vi "FM Voice Receiver.vi"() -> ()   [LabVIEW 2013]
uses:
  <vilib>/sound2/lvsound2.llb/Sound Output Write (DBL).vi
  <instrlib>/niUSRP/niUSRP Fetch Rx Data (CDB WDT).vi
  <vilib>/Analysis/2dsp.llb/Rational Resample (single channel, DBL).vi
  <vilib>/express/express analysis/Spectral/Block/exnSpectralBlock spectral measurements RMS poly.vi
  <vilib>/express/express analysis/Spectral/Block/exnSpectralBlock spectral measurements RMS WFM.vi
  <vilib>/express/express analysis/Spectral/XNode/ExpressSpectralMeasurementsBlockNode.xnode
  <vilib>/Analysis/NI_AALPro.lvlib
panel:
  out "File Error Out":errorcluster
  in  "Sound Format":T1={"sample rate (S/s)"=44100.0, "number of channels"=1.0, "bits per sample"=16.0}
  out "Spectrum (FFT)":cluster{"f0":dbl, "df":dbl, "magnitude":dbl[]}(graph)
  out "Waveform":waveform(dbl)(graph)
  out "Constellation":cluster{dbl[], dbl[]}(graph)
  out "USRP Error Out":errorcluster
  out "Coerced Gain":dbl format="%#_6f"
  out "Coerced Carrier Freq.":dbl=2400010000.007024 format="%#_6p"
  out "Coerced IQ Rate":dbl=200000.0 format="%#_6p"
  in  "Stop":bool
  in  "Active Antenna":string="RX2"
  in  "Gain":dbl format="%#_6f"
  in  "Carrier Frequency":dbl=1200000000.0 format="%#_6p"
  in  "IQ Rate":dbl=200000.0 format="%#_6p"
  in  "Device Address":refnum<k15>="192.168.10.2"
  in  "Number of Samples":i32=44100
  # "FM Receiver"
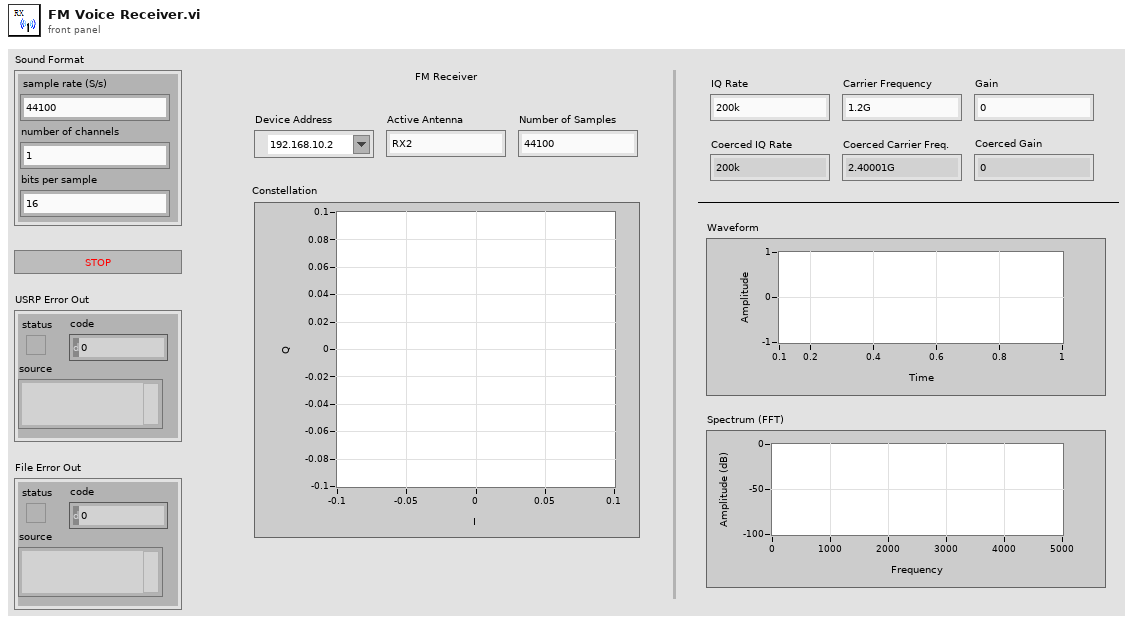
[diagram p1: front panel]
types:
  T1 = cluster{"sample rate (S/s)":dbl, "number of channels":dbl, "bits per sample":dbl}
  T2 = typedef "Sound Output Task ID.ctl" = u32
  T3 = cluster{"averaging mode":u16, "weighting mode":u16, "number of averages":u32}
  T4 = cluster{"dB On (F)":bool, "unwrap phase (F)":bool, "convert to degree (F)":bool}
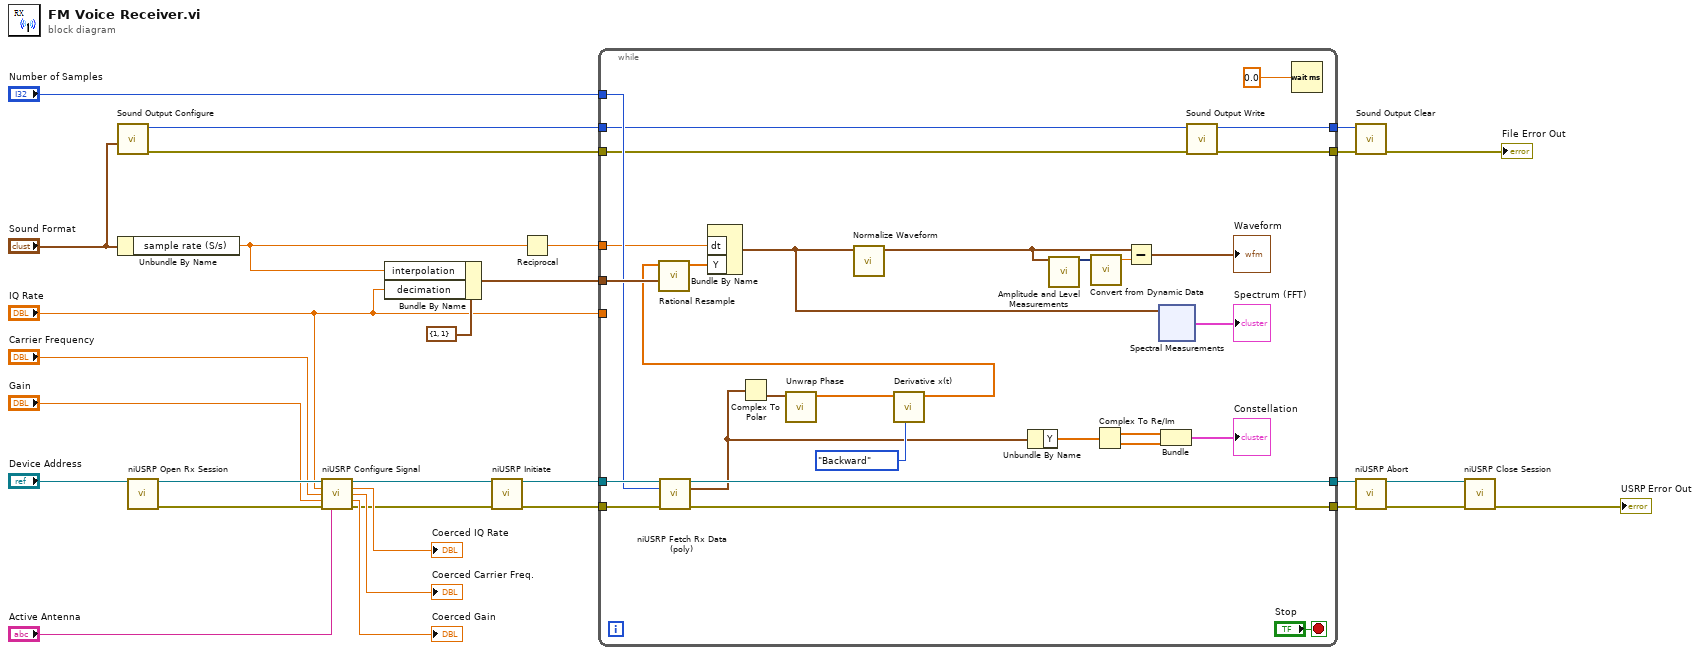
[diagram p0: block diagram]
diagram:
  n1 = call <vilib>:"Sound Output Configure.vi"("sound format"="Sound Format") -> ("error out"=w4:errorcluster, "task ID"=w5:T2)  [unwired: 9 in]
  n2 = Unbundle By Name("Sound Format") -> ("sample rate (S/s)"=w12:dbl)
  n3 = call <instrlib>:"niUSRP Open Rx Session.vi"("device names"="Device Address") -> ("session handle out"=w30:refnum<k15>, "error out"=w29:errorcluster)  [unwired: 13 in]
  n4 = call <instrlib>:"niUSRP Configure Signal.vi"("session handle"=w30, "IQ rate"="IQ Rate", "carrier frequency"="Carrier Frequency", "gain"="Gain", "error in (no error)"=w29, "active antenna"="Active Antenna") -> ("session handle out"=w16:refnum<k15>, "coerced IQ rate"=→"Coerced IQ Rate":dbl, "coerced carrier frequency"=→"Coerced Carrier Freq.":dbl, "coerced gain"=→"Coerced Gain":dbl, "error out"=w14:errorcluster)  [unwired: 5 in]
  n5 = Bundle By Name(cluster=cluster{"decimation":i32, "interpolation":i32} {"decimation"=1, "interpolation"=1}, "interpolation"=w12, "decimation"="IQ Rate") -> (w24:cluster{"decimation":i32, "interpolation":i32})
  n6 = call <instrlib>:"niUSRP Initiate.vi"("session handle"=w16, "error in (no error)"=w14) -> ("session handle out"=w15:refnum<k15>, "error out"=w13:errorcluster)  [unwired: 12 in]
  n7 = Reciprocal(x=w12) -> (1/x=w7:dbl)
  n8 = while {
    tunnel: w15 -> [w59]
    tunnel: [w57] -> w11
    tunnel: [w56] -> w10
    tunnel: w13 -> [w55]
    tunnel: "Number of Samples" -> [w51]
    tunnel: w24 -> [w54]
    tunnel: "IQ Rate" -> [_]
    tunnel: w7 -> [w45]
    tunnel: w5 -> [w40]
    tunnel: w4 -> [w39]
    tunnel: [w38] -> w3
    tunnel: [w37] -> w2
    stop <- "Stop" stop-if-true
    n9 = call-poly <instrlib>:"niUSRP Fetch Rx Data (poly).vi"("session handle"=w59, "number of samples"=w51, "error in (no error)"=w55) -> ("session handle out"=w57:refnum<k15>, "data"=w36:waveform(cdb), "error out"=w56:errorcluster)  [unwired: 9 in, 1 out]
    n10 = Complex To Polar(r * e^(i*theta)=w36) -> (theta=w44:waveform(dbl))  [unwired: 1 out]
    n11 = call <vilib>:"Unwrap Phase.vi"("Phase"=w44) -> ("Unwrapped Phase"=w43:dbl[])  [unwired: 9 in, 1 out]
    n12 = call <vilib>:"Derivative x(t).vi"("method"=enum16{"Backward"}."Backward", "X"=w43) -> ("dX/dt"=w41:dbl[])  [unwired: 8 in, 1 out]
    n13 = call-poly <vilib>:"Rational Resample.vi"("resample factor"=w54, "X"=w41) -> ("Y"=w46:dbl[])  [unwired: 7 in, 2 out]
    n14 = Bundle By Name("dt"=w45, "Y"=w46) -> (w32:waveform(dbl))  [unwired: 1 in]
    n15 = call <vilib>:"Normalize Waveform.vi"("waveform in"=w32) -> ("normalized waveform"=w35:waveform(dbl))  [unwired: 7 in, 3 out]
    n16 = Unbundle By Name(w36) -> ("Y"=w48:cdb[])
    n17 = call "Amplitude and Level Measurements"("Signals"=w35) -> ("Mean (DC)"=w34:dynamicdata)  [unwired: 13 in, 1 out]
    n18 = call "Convert from Dynamic Data"("Dynamic Data Type"=w34) -> ("Scalar"=w33:dbl)  [unwired: 3 in]
    n19 = Complex To Re/Im(x + iy=w48) -> (x=w50:dbl[], y=w49:dbl[])
    n20 = Subtract(x=w35, y=w33) -> (x-y=→"Waveform":waveform(dbl))
    n21 = xnode ("Spectral Measurements")("Signals"=w32) -> ("FFT - (RMS)"=→"Spectrum (FFT)":cluster{"f0":dbl, "df":dbl, "magnitude":dbl[]})  [unwired: 1 in, 2 out]
    n22 = Bundle(w50, w49) -> (→"Constellation":cluster{dbl[], dbl[]})  [unwired: 1 in]
    n23 = call-poly <vilib>:"Sound Output Write.vi"("error in (no error)"=w39, "task ID"=w40) -> ("error out"=w37:errorcluster, "task ID out"=w38:T2)  [unwired: 8 in]
    n24 = Wait (ms)(milliseconds to wait=0.0) -> ()  [unwired: 1 out]
  }
  n25 = call <vilib>:"Sound Output Clear.vi"("error in (no error)"=w2, "task ID"=w3) -> ("error out"=→"File Error Out":errorcluster)  [unwired: 9 in]
  n26 = call <instrlib>:"niUSRP Abort.vi"("session handle"=w11, "error in (no error)"=w10) -> ("session handle out"=w8:refnum<k15>, "error out"=w9:errorcluster)  [unwired: 12 in]
  n27 = call <instrlib>:"niUSRP Close Session.vi"("session handle"=w8, "error in (no error)"=w9) -> ("error out"=→"USRP Error Out":errorcluster)  [unwired: 13 in]
